vi "Dashboard Main.vi"() -> ()   [LabVIEW 2015]
uses:
  <vilib>/Utility/miscctls.llb/LVRowAndColumnTypeDef.ctl
  <vilib>/event_ctls.llb/eventvkey.ctl
  <vilib>/Rock Robotics/Network Tables/NT Read Numeric Array.vi
  <vilib>/Rock Robotics/WPI/Dashboard/WPI_DashboardLogging Global.vi
  Projects/FRC Operator Interface Control Board/controlBoard_LabVIEW/PWM_Output_TypeDef.ctl
  Projects/FRC Operator Interface Control Board/controlBoard_LabVIEW/LED_Output_TypeDef.ctl
  <vilib>/Rock Robotics/Network Tables/NT Write Raw.vi
  <vilib>/Rock Robotics/Network Tables/NT Read Raw.vi
panel:
  in  "TCP":refnum<k5>
  out "Image Message":string="Timeout in Camera Communications"
  in  "Dashboard Tab":T1(tab)
  out "Autonomous Selection":u8(ring) items=["Off", "Cross Defense", "Low Bar", "Cross Defense & Shoot", "Low Bar & Shoot"]
  out "Pneumatic Presure":u8(slide) scale=0.0..150.0
  out "Connected":bool
  out "COM Port":refnum<visa-resource-name>
  out "NT Connection":bool
  out "MotorChart R":cluster{"Numeric":dbl, "Numeric":dbl}(graph)
  out "MotorChart L":T2(graph)
  out "MotorSliders R":cluster{"MotorSlide1":dbl, "MotorSlide2":dbl} {"MotorSlide2" scale=-1.0..1.0 scale format="%#_2e"; "MotorSlide1" scale=-1.0..1.0 scale format="%#_2e"}
  out "MotorSliders L":T3 {"MotorSlide4 2" scale=0.0..14.0 scale format="%#_2e"; "MotorSlide2" scale=-1.0..1.0 scale format="%#_2e"; "MotorSlide1" scale=-1.0..1.0 scale format="%#_2e"}
  out "JS1 Z":dbl(slide) scale=-1.0..1.0 scale format="%#_2e"
  out "JS1 Graph":cluster{"X":dbl, "Y":dbl}[](graph)
  out "JS1 Buttons":T4
  out "JS2 Z":dbl(slide) scale=-1.0..1.0 scale format="%#_2e"
  out "JS2 Graph":cluster{"X":dbl, "Y":dbl}[](graph)
  out "JS2 Buttons":T4
  out "Mode":T5(ring)=enum."Auto Disabled"
  in  "DB Camera Config":bool
  out "fps":dbl format="%#.1g"
  out "Mbps":dbl format="%#.1g"
  out "Mbps LED":bool
  in  "Test Slider":dbl(slide) scale=0.0..100.0 scale format="%#_3g"
  in  "On/Off":bool caption="Solenoid"
  in  "Test Name":u16(ring) items=["Select the test to run..."]
  in  "Test Tree":string(tree)
  in  "Motor":cluster{"Value":dbl, "Enable":bool} {"Value" scale=-1.0..1.0 scale format="%#_3g"}
  out "Progress":T6 {"Test Progress" scale=0.0..100.0}
  in  "Rev/Fwd":cluster{"Forward":bool, "Reverse":bool}
  in  "Test Ring":u16(ring) items=["Monochrome", "Color"]
  out "Cmd Status":string
  in  "Execute Command":bool
  in  "Command Params":string[][](table)
  in  "Command Selection":i32(listbox)
  in  "CheckList":i32(listbox)
  out "Tree":string(tree)
  out "Camera Image":T7(plugin-control)
  # "Left"
  # "Front"
  # "Right"
  # "Battery"
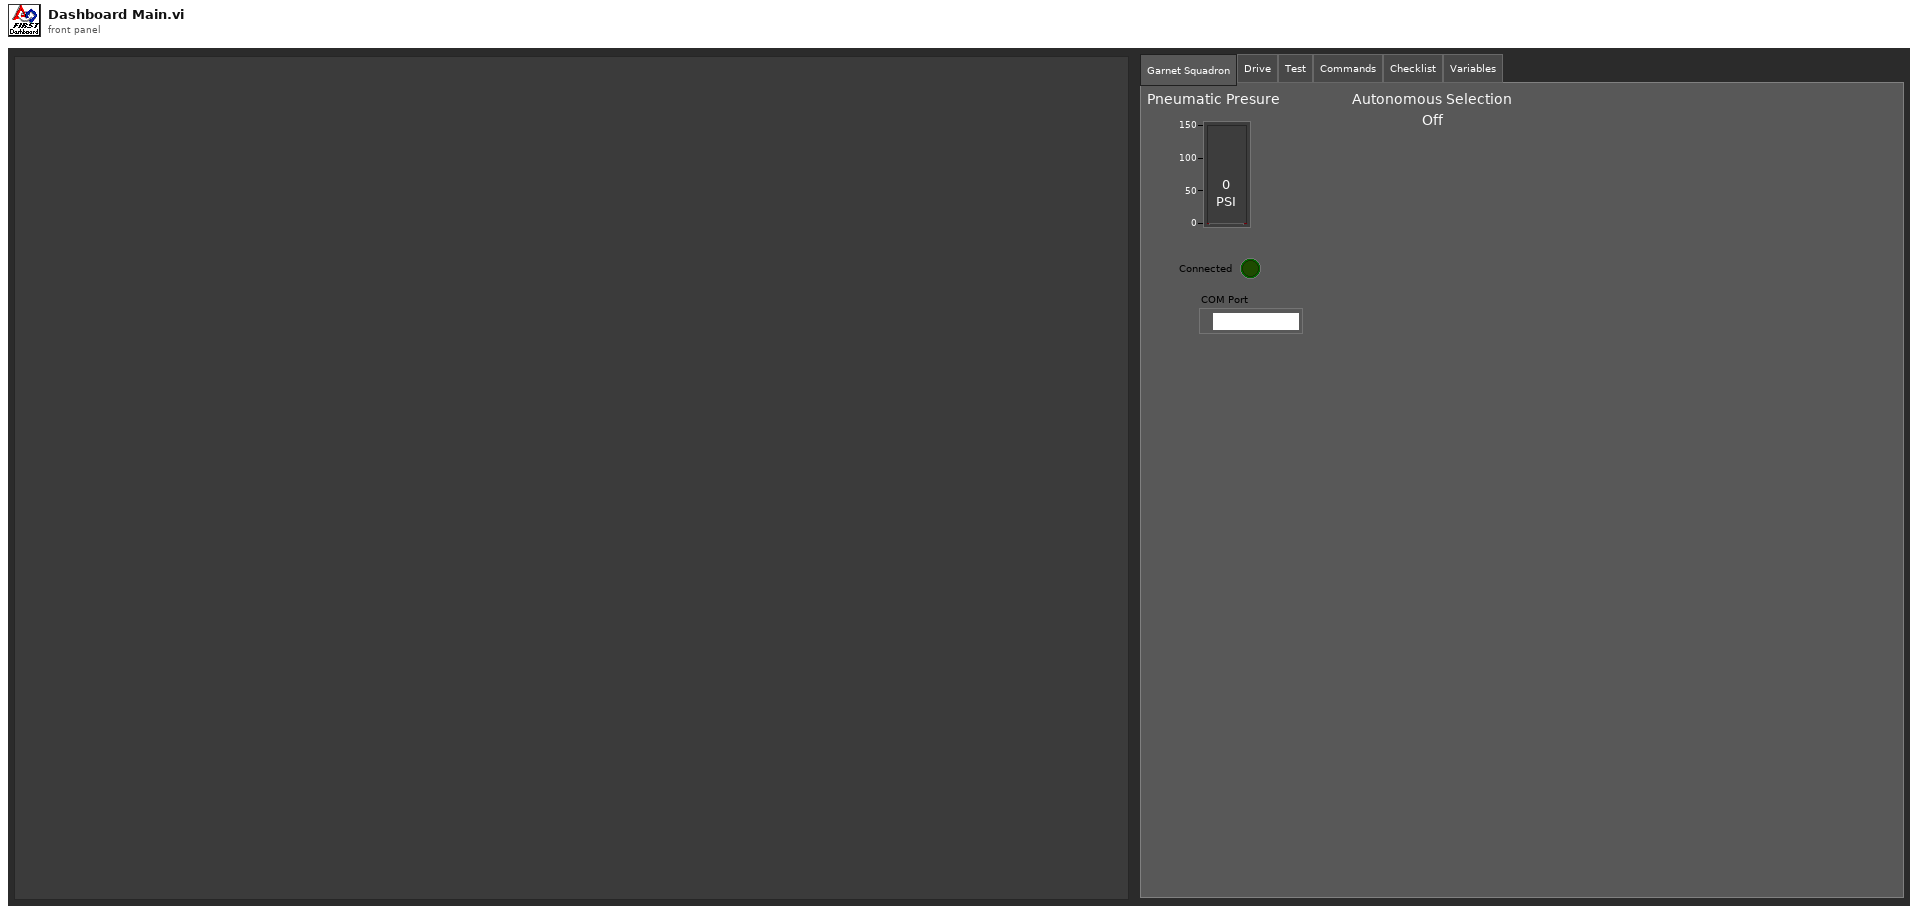
[diagram p1: front panel]
types:
  T1 = enum32{"Garnet Squadron", "Drive", "Test", "Commands", "Checklist", "Variables"}
  T2 = cluster{"Numeric":dbl, "Numeric":dbl, "Battery V":dbl}
  T3 = cluster{"MotorSlide1":dbl, "MotorSlide2":dbl, "MotorSlide4 2":dbl}
  T4 = cluster{bool, bool, bool, bool, bool, bool, bool, bool, bool, bool, bool, bool}
  T5 = enum8{"Tele-Op Disabled", "Tele-Op Enabled", "Auto Disabled", "Auto Enabled", "Test Disabled", "Test Enabled", "Disconnected", "No Code", "E-Stop"}
  T6 = cluster{"Test Progress":u8, "Test Progress Text":string}
  T7 = typedef "IMAQ Image.ctl" = refnum<image>
  T8 = enum8{"Enabled", "Disabled", "Disabled and Grayed Out"}
  T9 = cluster{"IDs":cluster{"RPC field ID":u16, "Unique ID":u16}, "String":string}
  T10 = enum32{"Drive", "Basic", "Custom", "Test", "Checklist", "Variables"}
  T11 = typedef "Image Type" = u32
  T12 = typedef "LED_Output_TypeDef.ctl" = cluster{"LED 0":bool, "LED 1":bool, "LED 2":bool, "LED 3":bool, "LED 4":bool, "LED 5":bool, "LED 6":bool, "LED 7":bool, "LED 8":bool, "LED 9":bool, "LED 10":bool, "LED 11":bool, "LED 12":bool, "LED 13":bool, "LED 14":bool, "LED 15":bool}
  T13 = typedef "PWM_Output_TypeDef.ctl" = cluster{"PWM 0":u8, "PWM 1":u8, "PWM 2":u8, "PWM 3":u8, "PWM 4":u8, "PWM 5":u8, "PWM 6":u8, "PWM 7":u8, "PWM 8":u8, "PWM 9":u8, "PWM 10":u8}
  T14 = typedef "Analog_Input_TypeDef.ctl" = cluster{"ANA 0":u8, "ANA 1":u8, "ANA 2":u8, "ANA 3":u8, "ANA 4":u8, "ANA 5":u8, "ANA 6":u8, "ANA 7":u8, "ANA 8":u8, "ANA 9":u8, "ANA 10":u8, "ANA 11":u8, "ANA 12":u8, "ANA 13":u8, "ANA 14":u8, "ANA 15":u8}
  T15 = typedef "Switch_Input_TypeDef.ctl" = cluster{"SW 0":bool, "SW 1":bool, "SW 2":bool, "SW 3":bool, "SW 4":bool, "SW 5":bool, "SW 6":bool, "SW 7":bool, "SW 8":bool, "SW 9":bool, "SW 10":bool, "SW 11":bool, "SW 12":bool, "SW 13":bool, "SW 14":bool, "SW 15":bool}
  T16 = cluster{"Error Strings":string, "Disable Counts":cluster{u16, u16}, "Rail Faults":cluster{u16, u16, u16}, "Robot IP":string, "DB Mode":u8, "Event Info":cluster{"Name":string, "Type":u8, "Number":u16, "Replay":u8}, "Camera Addr":string}
  T17 = cluster{"Storage":cluster{"Disk Free":u64, "RAM Block":u32, "RAM free":u32}, "CPU Utilization":cluster{"CPU % ISR":sgl, "CPU % Time Crit":sgl, "CPU % Timed Str":sgl, "CPU % High":sgl, "CPU % Above":sgl, "CPU % Normal":sgl, "CPU % Low":sgl}, "CAN":cluster{"% Bus Utilization":sgl, "Bus Off Cnt":u32, "TX_FIFO Full Cnt":u32, "Receive Error Cnt":u8, "Transmit Error Cnt":u8}, "HID":cluster{"HID Outputs":u32, "Rumble Low":u16, "Rumble High":u16}[]}
  T18 = cluster{"Status bits":cluster{"Test Mode":bool, "Autonomous":bool, "Enabled":bool, "Code Start":bool, "Brownout":bool, "Reserved 2":bool, "Reserved 3":bool, "E-Stop":bool}, "Code Trace":cluster{"Disabled":bool, "TeleOp":bool, "Auto":bool, "Test":bool}, "Controller Type":enum16{"unknown", "cRIO", "roboRio"}, "Code?":enum16{"unknown", "noCode", "code"}, "Battery V":dbl}
  T19 = cluster{"Control Bits":cluster{"TestMode":bool, "Autonomous":bool, "Enabled":bool, "FMS Present":bool, bool, bool, bool, "E-Stop":bool}, "Team Station ":u8, "Countdown":sgl, "Joystick Values":cluster{"Axes":dbl[], "Buttons":bool[], "POVs":i16[]}[]}
  T20 = cluster{"Axes":dbl[], "Buttons":bool[], "POVs":i16[]}[]
  T21 = cluster{"Axes":dbl[], "Buttons":bool[], "POVs":i16[]}
  T22 = cluster{"Buttons[0]":bool, "Buttons[1]":bool, "Buttons[2]":bool, "Buttons[3]":bool, "Buttons[4]":bool, "Buttons[5]":bool, "Buttons[6]":bool, "Buttons[7]":bool, "Buttons[8]":bool, "Buttons[9]":bool, "Buttons[10]":bool, "Buttons[11]":bool}
  T23 = typedef "NI_LVConfig.lvlib/Config Data RefNum.ctl" = refnum<k1>
  T24 = cluster{"Operation":enum16{"Update", "Clear"}, "Color Box":u32}[]
  T25 = typedef "eventvkey.ctl" = enum16{"ASCII", "Enter", "Return", "Shift", "Ctrl", "Alt", "Cmd", "Opt", "Caps", "NumLock", "Clear", "Break", "Up", "Down", "Left", "Right", "Insert", "Delete", "Home", "End", "PageUp", "PageDown", "Escape", "Help", "Pause", "ScrollLock", "F1", "F2", "F3", "F4", "F5", "F6", "F7", "F8", "F9", "F10", "F11", "F12", "F13", "F14", "F15", "F16", "F17", "F18", "F19", "F20", "F21", "F22", "F23", "F24", "Play", "VolumeUp", "VolumeDown", "Mute", "Two Byte Char"}
  T26 = cluster{"Operation":enum16{"Update", "Clear"}, "Color Box":u32}
  T27 = typedef "LVRowAndColumnTypeDef.ctl" = cluster{"Row":i32, "Column":i32}
  T28 = cluster{"Shift":bool, "Ctrl":bool, "Alt":bool, "Cmd":bool, "Opt":bool}
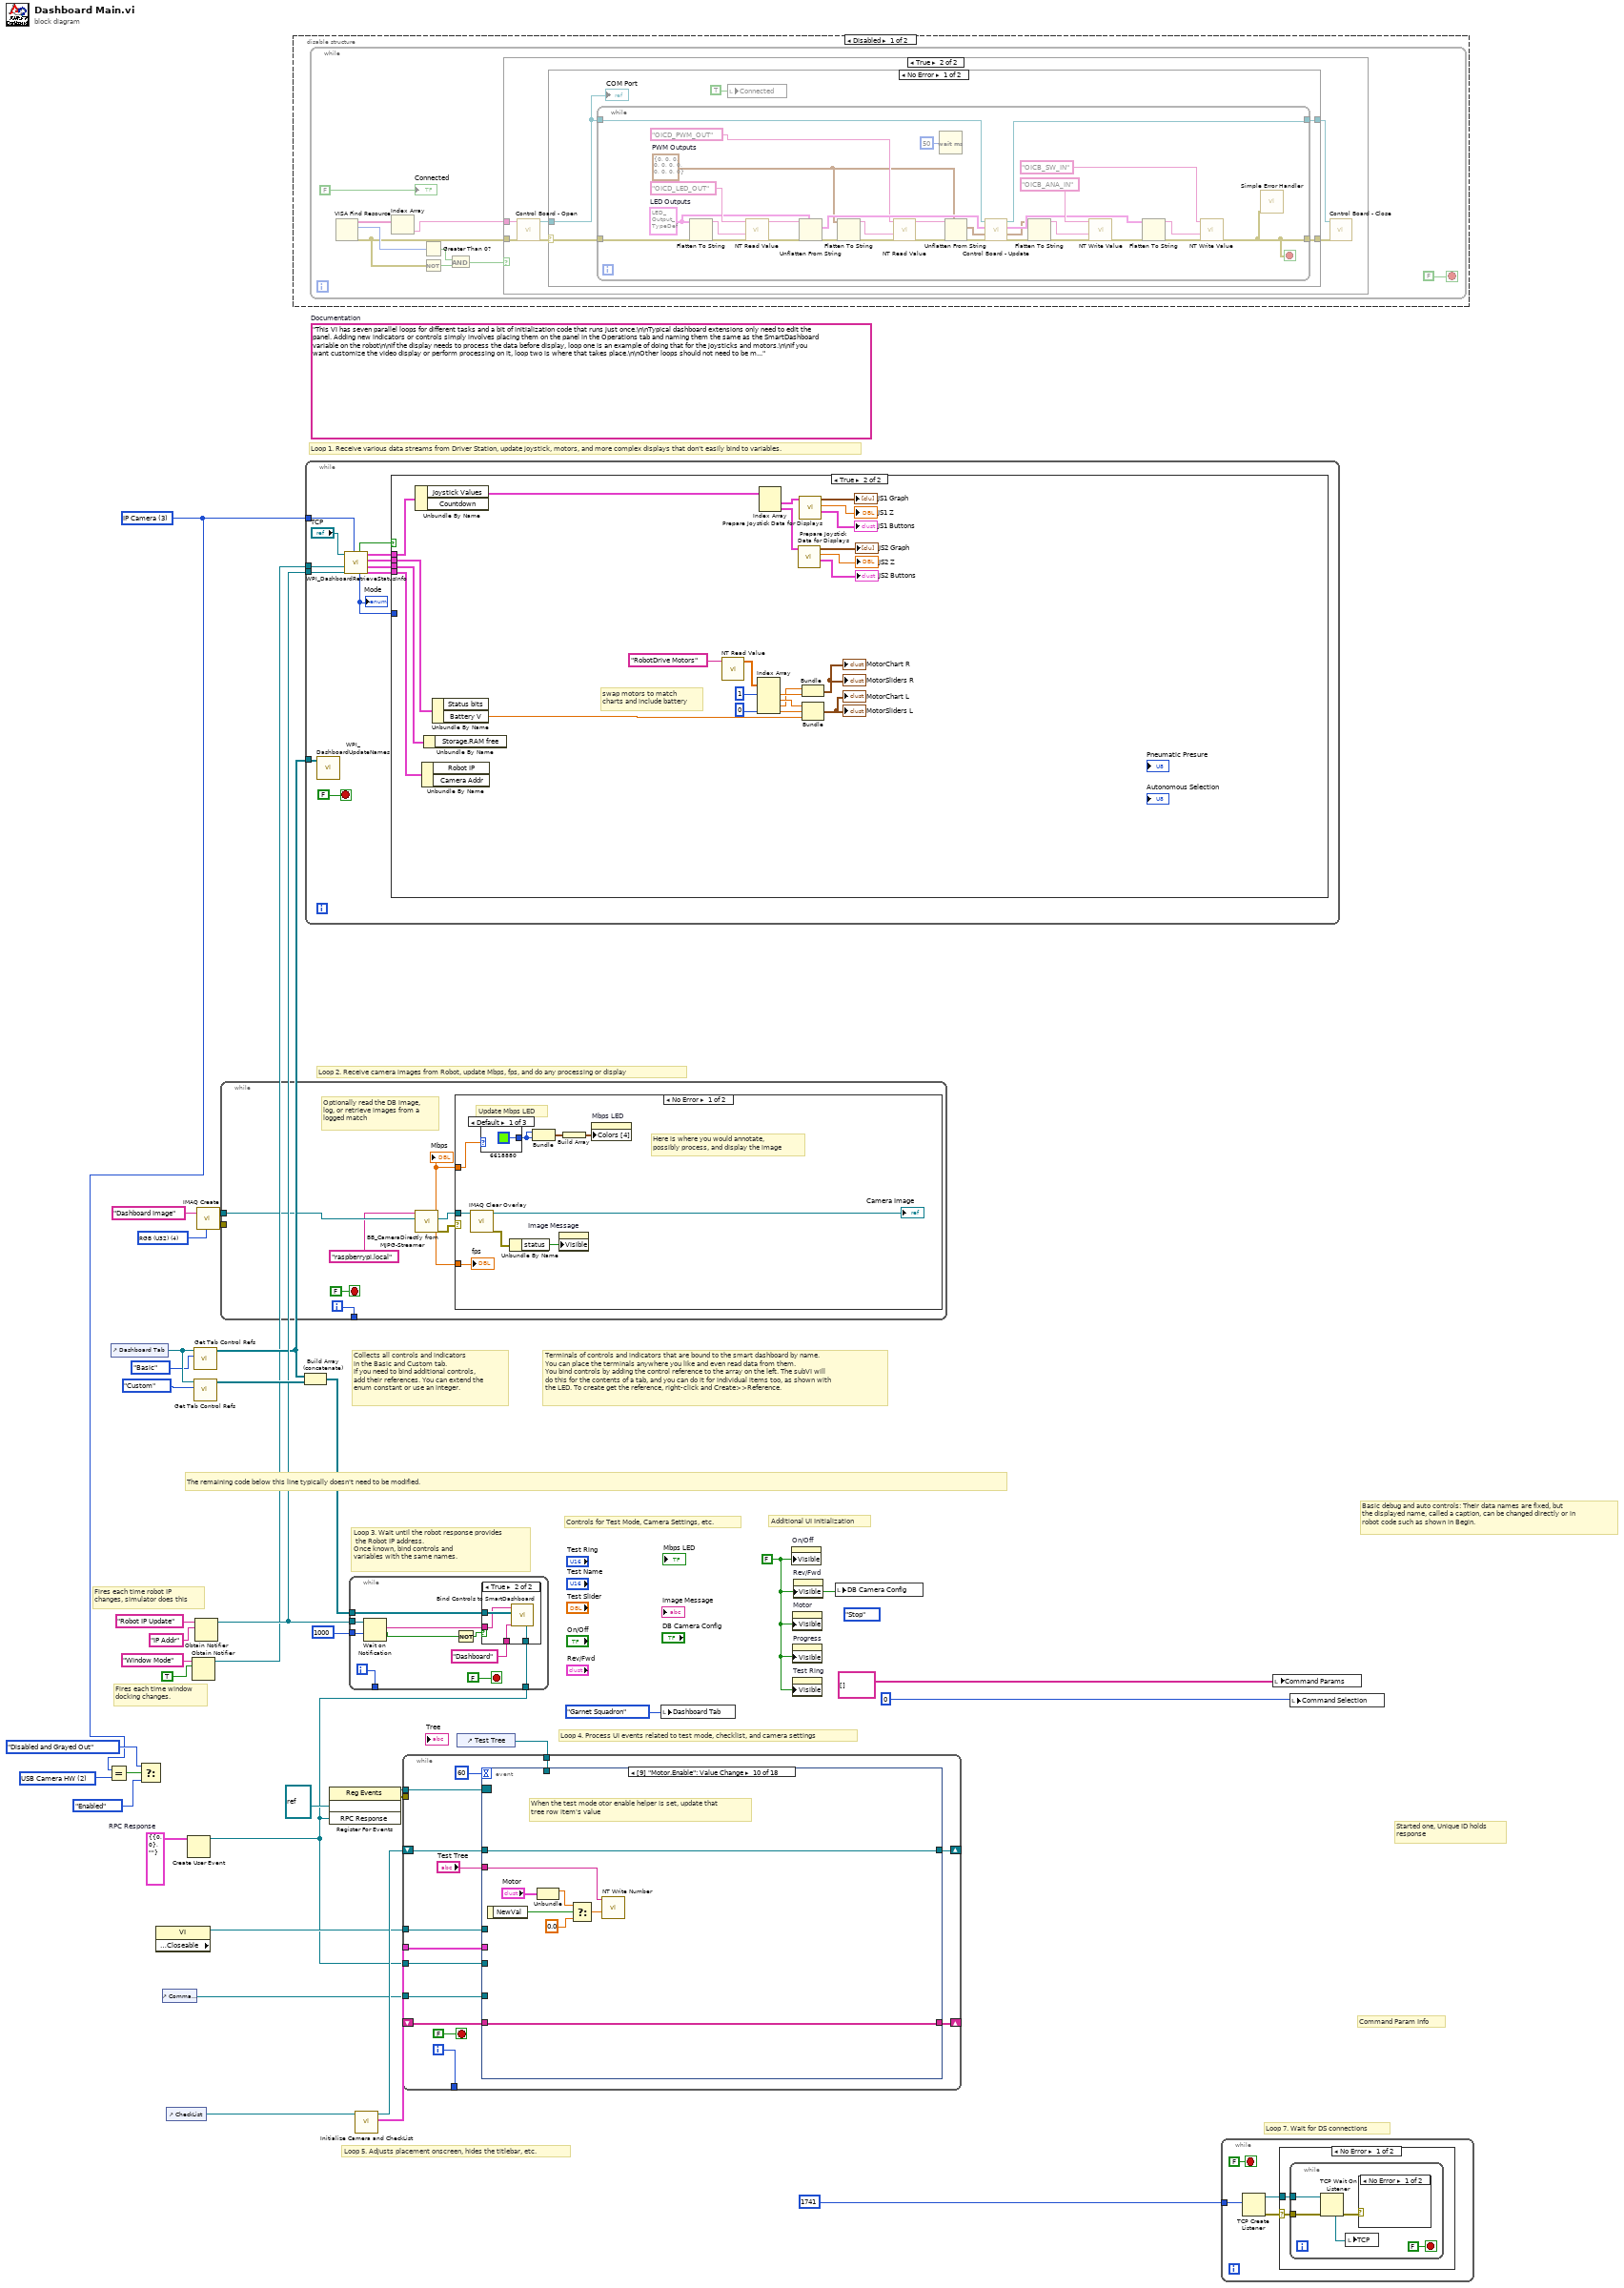
[diagram p0: block diagram]
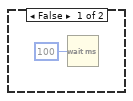
[diagram p2: hidden frame]
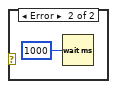
[diagram p5: hidden frame]
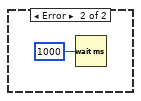
[diagram p6: hidden frame]
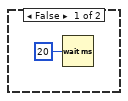
[diagram p7: hidden frame]
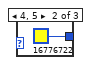
[diagram p9: hidden frame]
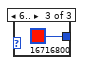
[diagram p10: hidden frame]
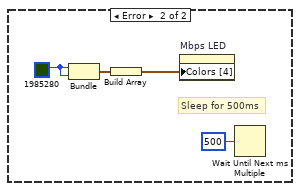
[diagram p11: hidden frame]
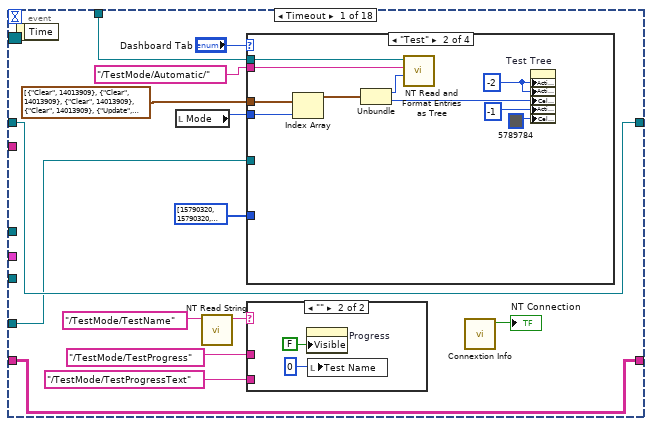
[diagram p12: hidden frame]
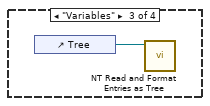
[diagram p14: hidden frame]
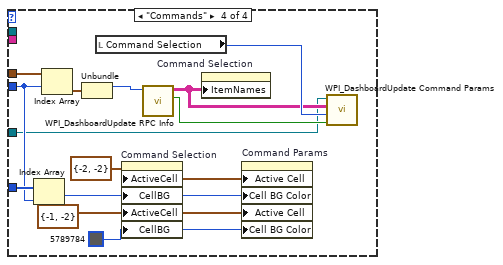
[diagram p15: hidden frame]
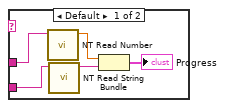
[diagram p16: hidden frame]
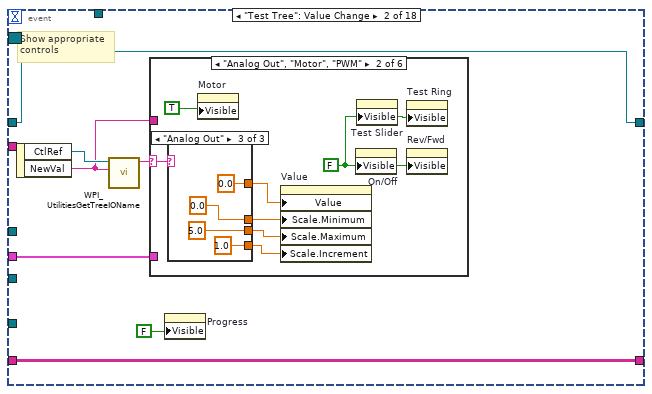
[diagram p17: hidden frame]
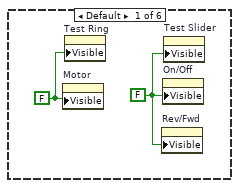
[diagram p18: hidden frame]
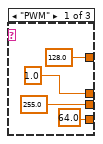
[diagram p19: hidden frame]
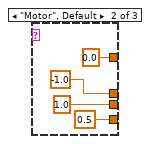
[diagram p20: hidden frame]
diagram:
  w1 = u16 2 items=["Camera Off", "USB Camera SW", "USB Camera HW", "IP Camera"] ("Vision")
  w2 = u16 3 items=["Camera Off", "USB Camera SW", "USB Camera HW", "IP Camera"] ("Vision")
  w10 = T9 {"IDs"={"RPC field ID"=0, "Unique ID"=0}, "String"=""}  # RPC Response
  (unwired) enum32{"Stop", "Record", "Playback"}."Stop" ("Rec Mode")
  w16 = FALSE ("Visible")
  (unwired) "This VI has seven parallel loops for different tasks and a bit of initialization code that runs just once.\n\nTypical dashboard extensions only need to edit the panel. Adding new indicators or controls simply involves placing them on the panel in the Operations tab and naming them the same as the SmartDashboard variable on the robot\n\nIf the display needs to process the data before display, loop one is an example of doing that for the joysticks and motors.\n\nIf you want customize the video display or perform processing on it, loop two is where that takes place.\n\nOther loops should not need to be modified. They are pretty standard, and document the task they perform."  # Documentation
  w38 = T11 4 items=["Grayscale (U8)", "Grayscale (I16)", "Grayscale (SGL)", "Complex (CSG)", "RGB (U32)", "HSL (U32)", "RGB (U64)"] ("Image Type")
  # "Command Param Info"
  # "Started one, Unique ID holds\nresponse"
  # "Loop 7. Wait for DS connections"
  # "Basic debug and auto controls: Their data names are fixed, but\nthe displayed name, called a caption, can be changed directly or in\nrobot code such as shown in Begin."
  # "Controls for Test Mode, Camera Settings, etc."
  # "Additional UI Initialization"
  # "Fires each time robot IP\nchanges, simulator does this"
  # "Fires each time window\ndocking changes."
  # "Collects all controls and indicators\nin the Basic and Custom tab.\nIf you need to bind additional controls,\nadd their references. You can extend the\nenum constant or use an integer."
  # "The remaining code below this line typically doesn't need to be modified."
  # "Loop 4. Process UI events related to test mode, checklist, and camera settings"
  # "Terminals of controls and indicators that are bound to the smart dashboard by name.\nYou can place the terminals anywhere you like and even read data from them.\nYou bind controls by adding the control reference to the array on the left. The subVI will\ndo this for the contents of a tab, and you can do it for individual items too, as shown with\nthe LED. To create get the reference, right-click and Create>>Reference."
  # "Loop 3. Wait until the robot response provides\n the Robot IP address.\nOnce known, bind controls and\nvariables with the same names."
  # "Loop 5. Adjusts placement onscreen, hides the titlebar, etc."
  # "Loop 1. Receive various data streams from Driver Station, update joystick, motors, and more complex displays that don't easily bind to variables."
  # "Loop 2. Receive camera images from Robot, update Mbps, fps, and do any processing or display"
  n1 = Equal?(x=w2, y=w1) -> (x = y?=w5:bool)
  n2 = control-ref of="Dashboard Tab"() -> (w22:refnum<vi>)
  n3 = Select(t=T8."Disabled and Grayed Out" ("Disabled"), s=w5, f=T8."Enabled" ("Disabled")) -> ()  [unwired: 1 out]
  n4 = property class="VI" props=["Front Panel.Closeable"]() -> (reference out=w23:refnum<vi>)  [unwired: 2 in, 2 out]
  n5 = control-ref of="Command Params"() -> (w6:refnum<vi>)
  n6 = control-ref of="CheckList"() -> (w17:refnum<vi>)
  n7 = Create User Event(user event datatype=w10) -> (user event=w7:refnum<user-event>)  [unwired: 1 in, 1 out]
  n8 = Obtain Notifier(name (unnamed)="Window Mode", notification data type=TRUE) -> (notifier out=w13:refnum<notifier>)  [unwired: 2 in, 2 out]
  n9 = call <vilib>:"Get Tab Control Refs.vi"("Page Index"=T10."Basic" ("Dashboard Tab"), "TabControl in"=w22) -> ("ControlsOnPage"=w14:refnum<vi>[])  [unwired: 9 in]
  n10 = call <vilib>:"Get Tab Control Refs.vi"("Page Index"=T10."Custom" ("Dashboard Tab"), "TabControl in"=w22) -> ("ControlsOnPage"=w21:refnum<vi>[])  [unwired: 9 in]
  n11 = Obtain Notifier(name (unnamed)="Robot IP Update", notification data type="IP Addr" ("name (unnamed)")) -> (notifier out=w15:refnum<notifier>)  [unwired: 2 in, 2 out]
  n12 = call "IMAQ Create"("Image Name"="Dashboard Image", "Image Type"=w38) -> ("New Image"=w36:T7, "error out"=w35:errorcluster)  [unwired: 2 in, 1 out]
  n13 = while {
    tunnel: w36 -> [w44]
    tunnel: w35 -> [_]
    tunnel: [w45] -> _
    i -> [w45]
    stop <- FALSE stop-if-true
    # "Optionally read the DB image,\nlog, or retrieve images from a\nlogged match"
    n14 = call "BB_CameraDirectly from MJPG-Streamer.vi"("Image"=w44, "address"="raspberrypi.local" ("Camera IP")) -> ("error out"=w42:errorcluster, "Bandwidth (Mbps)"=w40:dbl, "Image Out"=w43:T7, "FPS"=w41:dbl)  [unwired: 6 in]
    "Mbps" <- w40
    n15 = case shown="No Error" w42 {
      tunnel: w43 -> [w50 _]
      tunnel: w40 -> [w49 _]
      tunnel: w41 -> [w47 _]
      frame No Error {
        # "Here is where you would annotate,\npossibly process, and display the image"
        # "Update Mbps LED"
        n16 = call "IMAQ Clear Overlay"("Image"=w50) -> ("error out"=w54:errorcluster, "Image Out"=→"Camera Image":T7)  [unwired: 2 in, 7 out]
        n17 = case shown="Default" w49 {
          tunnel: [u32 6618880 ("Color Box") u32 16776722 ("Color Box") u32 16716800 ("Color Box")] -> w51
          frame Default {
          }
          frame 4, 5 {
          }
          frame 6.. {
          }
        }
        n18 = Unbundle By Name(w54) -> ("status"=w55:bool)
        n19 = Bundle("Color Box"=w51, "Color Box"=w51) -> (w53:cluster{"Color Box":u32, "Color Box":u32})  [unwired: 1 out]
        n20 = property on="Image Message" class="Str"("Visible"=w55) -> ()  [unwired: 2 in, 2 out]
        n21 = Build Array(w53) -> (w52:cluster{"Color Box":u32, "Color Box":u32}[])
        n22 = property on="Mbps LED" class="Bool (strict)"("Colors [4]"=w52) -> ()  [unwired: 2 in, 2 out]
        "fps" <- w47
      }
      frame Error {
        w59 = u32 1985280 ("Color Box")
        # "Sleep for 500ms"
        n23 = Bundle("Color Box"=w59, "Color Box"=w59) -> (w61:cluster{"Color Box":u32, "Color Box":u32})  [unwired: 1 out]
        n24 = Build Array(w61) -> (w60:cluster{"Color Box":u32, "Color Box":u32}[])
        n25 = property on="Mbps LED" class="Bool (strict)"("Colors [4]"=w60) -> ()  [unwired: 2 in, 2 out]
        n26 = Wait Until Next ms Multiple(millisecond multiple=u32 500) -> ()  [unwired: 1 out]
      }
    }
  }
  n27 = disable-structure shown="Disabled" {
    frame Disabled {
      n28 = while {
        stop <- FALSE stop-if-true
        n29 = VISA Find Resource() -> (0:w65:errorcluster, 2:w71:u32, 3:w70:string[])  [unwired: 3 in]
        n30 = Index Array(array=w70) -> (element=w69:string)  [unwired: 1 in]
        n31 = Greater Than 0?(x=w71) -> (x > 0?=w68:bool)
        n32 = Not(x=w65) -> (.not. x?=w66:bool)
        n33 = And(x=w68, y=w66) -> (x .and. y?=w67:bool)
        n34 = case shown="True" w67 {
          tunnel: w69 -> [_ w77]
          tunnel: w65 -> [_ w76]
          frame False {
            n35 = Wait (ms)(milliseconds to wait=u32 100) -> ()  [unwired: 1 out]
          }
          frame True {
            n36 = call "Control Board - Open.vi"("error in (no error)"=w76, "VISA Refnum in"=w77) -> ("error out"=w75:errorcluster, "VISA Refnum out"=w78:refnum<visa-resource-name>)  [unwired: 8 in]
            n37 = case shown="No Error" w75 {
              selector: w75 -> [w82 w116]
              tunnel: w78 -> [w83 w115]
              tunnel: [w80 w116] -> w74
              tunnel: [w79 w115] -> w73
              frame No Error {
                n38 = while {
                  tunnel: w83 -> [w114]
                  tunnel: [w112] -> w79
                  tunnel: [w84] -> w80
                  tunnel: w82 -> [w86]
                  stop <- w84 stop-if-true
                  w93 = T12 {"LED 0"=FALSE, "LED 1"=FALSE, "LED 2"=FALSE, "LED 3"=FALSE, "LED 4"=FALSE, "LED 5"=FALSE, "LED 6"=FALSE, "LED 7"=FALSE, "LED 8"=FALSE, "LED 9"=FALSE, "LED 10"=FALSE, "LED 11"=FALSE, "LED 12"=FALSE, "LED 13"=FALSE, "LED 14"=FALSE, "LED 15"=FALSE}  # LED Outputs
                  w91 = T13 {"PWM 0"=0, "PWM 1"=0, "PWM 2"=0, "PWM 3"=0, "PWM 4"=0, "PWM 5"=0, "PWM 6"=0, "PWM 7"=0, "PWM 8"=0, "PWM 9"=0, "PWM 10"=0}  # PWM Outputs
                  n39 = Flatten To String(anything=w93, error in (no error)=w86) -> (data string=w92:string, error out=w87:errorcluster)  [unwired: 2 in, 1 out]
                  n40 = call-poly <vilib>:"NT Read Value.vi"("error in"=w87, "Default Value"=w92, "Name"="OICD_LED_OUT") -> ("error out"=w100:errorcluster, "Raw"=w102:string)  [unwired: 7 in]
                  n41 = Unflatten From String(type=w93, binary string=w102, error in (no error)=w100) -> (value=w104:T12, error out=w88:errorcluster)  [unwired: 2 in, 1 out]
                  n42 = Flatten To String(anything=w91, error in (no error)=w88) -> (data string=w90:string, error out=w89:errorcluster)  [unwired: 2 in, 1 out]
                  n43 = call-poly <vilib>:"NT Read Value.vi"("error in"=w89, "Default Value"=w90, "Name"="OICD_PWM_OUT") -> ("error out"=w95:errorcluster, "Raw"=w108:string)  [unwired: 7 in]
                  n44 = Wait (ms)(milliseconds to wait=u32 50) -> ()  [unwired: 1 out]
                  n45 = Unflatten From String(type=w91, binary string=w108, error in (no error)=w95) -> (value=w107:T13, error out=w94:errorcluster)  [unwired: 2 in, 1 out]
                  n46 = call "Control Board - Update.vi"("error in (no error)"=w94, "PWM Outputs"=w107, "LED Outputs"=w104, "Control Board VISA Reference In"=w114) -> ("error out"=w97:errorcluster, "Analog Inputs"=w106:T14, "Switch Inputs"=w110:T15, "Control Board VISA Reference Out"=w112:refnum<visa-resource-name>)  [unwired: 4 in]
                  n47 = Flatten To String(anything=w106, error in (no error)=w97) -> (data string=w105:string, error out=w99:errorcluster)  [unwired: 2 in, 1 out]
                  n48 = call-poly <vilib>:"NT Write Value.vi"("error in"=w99, "Raw"=w105, "Name"="OICB_ANA_IN") -> ("error out"=w96:errorcluster)  [unwired: 8 in]
                  n49 = Flatten To String(anything=w110, error in (no error)=w96) -> (data string=w109:string, error out=w98:errorcluster)  [unwired: 2 in, 1 out]
                  n50 = call-poly <vilib>:"NT Write Value.vi"("error in"=w98, "Raw"=w109, "Name"="OICB_SW_IN") -> ("error out"=w84:errorcluster)  [unwired: 8 in]
                  n51 = call <vilib>:"Simple Error Handler.vi"("error in (no error)"=w84) -> ()  [unwired: 4 in, 5 out]
                }
                n52 = local write "Connected"(TRUE ("Connected")) -> ()
                "COM Port" <- w83
              }
              frame Error {
              }
            }
            n53 = call "Control Board - Close.vi"("error in (no error)"=w74, "VISA Refnum in"=w73) -> ()  [unwired: 9 in, 1 out]
          }
        }
        "Connected" <- FALSE
      }
    }
    frame Enabled {
    }
  }
  n54 = Build Array (concatenate)(w14, w21) -> (w20:refnum<vi>[])
  n55 = while {
    tunnel: w15 -> [w122]
    tunnel: w14 -> [w121]
    tunnel: w13 -> [w118]
    tunnel: w2 -> [w117]
    stop <- FALSE stop-if-true
    n56 = call <vilib>:"WPI_DashboardUpdateNames.vi"("Controls on Tab"=w121) -> ()  [unwired: 11 in]
    n57 = call <vilib>:"WPI_DashboardRetrieveStatusInfo.vi"("Vision"=w117, "Binding Refnum"=w122, "Window Mode Notifier"=w118, "TCP Cnx"="TCP") -> ("Power and Errors"=w123:T16, "Robot Metrics"=w126:T17, "Status Info"=w127:T18, "Control Info"=w124:T19, "Robot Mode"=w120:T5, "Process?"=w125:bool)  [unwired: 2 in]
    "Mode" <- w120
    n58 = case shown="True" w125 {
      tunnel: w127 -> [_ w153]
      tunnel: w126 -> [_ w152]
      tunnel: w124 -> [_ w151]
      tunnel: w123 -> [_ w150]
      tunnel: w120 -> [_ _]
      frame False {
        n59 = Wait (ms)(milliseconds to wait=u32 20) -> ()  [unwired: 1 out]
      }
      frame True {
        # "swap motors to match\ncharts and include battery"
        n60 = Unbundle By Name(w151) -> ("Joystick Values"=w140:T20)  [unwired: 1 out]
        n61 = Unbundle By Name(w150) -> ()  [unwired: 2 out]
        n62 = Unbundle By Name(w152) -> ()  [unwired: 1 out]
        n63 = Unbundle By Name(w153) -> ("Battery V"=w141:dbl)  [unwired: 1 out]
        n64 = call-poly <vilib>:"NT Read Value.vi"("Name"="RobotDrive Motors") -> ("Numeric Array"=w130:dbl[])  [unwired: 9 in, 1 out]
        n65 = Index Array(array=w130, index #1=1, index #4=0) -> (element #1=w145:dbl, element #2=w146:dbl, element #3=w144:dbl, element #4=w149:dbl)  [unwired: 2 in]
        n66 = Index Array(array=w140) -> (element #1=w139:T21, element #2=w135:T21)  [unwired: 2 in]
        n67 = call "Prepare Joystick Data for Displays.vi"("Joystick Values"=w135) -> ("Buttons"=→"JS2 Buttons":T22, "Z Axis"=→"JS2 Z":dbl, "Cartesian Data"=→"JS2 Graph":cluster{"X axis":dbl, "X axis":dbl}[])  [unwired: 8 in]
        n68 = call "Prepare Joystick Data for Displays.vi"("Joystick Values"=w139) -> ("Buttons"=→"JS1 Buttons":T22, "Z Axis"=→"JS1 Z":dbl, "Cartesian Data"=→"JS1 Graph":cluster{"X axis":dbl, "X axis":dbl}[])  [unwired: 8 in]
        n69 = Bundle("Numeric"=w144, "Numeric"=w145) -> (→"MotorChart R" →"MotorSliders R":cluster{"Numeric":dbl, "Numeric":dbl})  [unwired: 1 in]
        n70 = Bundle("Numeric"=w146, "Numeric"=w149, "Battery V"=w141) -> (→"MotorChart L" →"MotorSliders L":T2)  [unwired: 1 in]
      }
    }
  }
  n71 = register-events(refnum<vi> refnum, w7) -> (reference out=w27:refnum<event-registration>, error out=w26:errorcluster)  [unwired: 2 in]
  n72 = while {
    tunnel: w20 -> [w163]
    tunnel: w15 -> [w161]
    tunnel: [w159] -> _
    tunnel: u32 1000 ("milliseconds to wait") -> [w158]
    tunnel: w7 -> [w154]
    i -> [w159]
    stop <- FALSE stop-if-true
    n73 = Wait on Notification(notifier=w161, timeout in ms (-1)=w158) -> (notification=w160:string, timed out?=w156:bool)  [unwired: 2 in, 2 out]
    n74 = Not(x=w156) -> (.not. x?=w157:bool)
    n75 = case shown="True" w157 {
      tunnel: w163 -> [_ w167]
      tunnel: w160 -> [_ w166]
      tunnel: "Dashboard" -> [_ w165]
      tunnel: w154 -> [_ w164]
      frame False {
      }
      frame True {
        n76 = call <vilib>:"Bind Controls to SmartDashboard.vi"("RPC ref"=w164, "Client Name"=w165, "Bound Control Refs"=w167, "Server IP Address"=w166) -> ()  [unwired: 8 in]
      }
    }
  }
  n77 = call "Initialize Camera and CheckList.vi"("ListBox in"=w17) -> ("Array"=w30:cluster{string[]}[], "File Refnum"=w29:T23)  [unwired: 8 in, 1 out]
  n78 = control-ref of="Test Tree"() -> (w28:refnum<vi>)
  n79 = while {
    tunnel: w30 -> [w178]
    shift-right: [w177] -> _
    shift-left: w29 -> [w176]
    tunnel: [w175] -> _
    tunnel: w28 -> [w174]
    tunnel: w27 -> [w173]
    tunnel: w26 -> [_]
    tunnel: w23 -> [w172]
    tunnel: w7 -> [w171]
    tunnel: w6 -> [w170]
    shift-right: [w169] -> _
    shift-left: _ -> [w168]
    i -> [w175]
    stop <- FALSE stop-if-true
    n80 = event shown="[9] \"Motor.Enable\": Value Change" {
      selector: w173 -> [_ _ _ _ _ _ _ _ _ _ _ _ _ _ _ _ _ _]
      dyn-events: _ -> [_ _ _ _ _ _ _ _ _ _ _ _ _ _ _ _ _ _]
      timeout: u32 60 ("milliseconds to wait") -> [_ _ _ _ _ _ _ _ _ _ _ _ _ _ _ _ _ _]
      tunnel: w174 -> [w191 _ _ _ _ _ _ _ _ _ _ _ _ _ _ _ _ _]
      tunnel: "Test Tree" -> [_ _ _ _ _ _ _ _ _ w403 w412 w415 w420 w429 _ _ _ _]
      tunnel: w178 -> [_ w229 _ _ _ _ _ _ _ _ _ _ _ _ _ _ _ _]
      tunnel: [w188 w228 w332 w338 w350 w362 w370 w376 w389 w402 w410 w414 w419 w428 w435 w437 w444 w452] -> w177
      tunnel: w176 -> [w188 w228 w332 w338 w350 w362 w370 w376 w389 w402 w410 w414 w419 w428 w435 w437 w444 w452]
      tunnel: w172 -> [_ _ _ _ _ _ _ _ _ _ _ _ _ _ _ _ _ _]
      tunnel: w171 -> [_ _ _ _ _ _ _ _ _ _ _ _ _ _ _ _ _ _]
      tunnel: w170 -> [w183 _ _ _ w348 _ _ _ _ _ _ _ _ _ _ _ _ _]
      tunnel: [w182 w227 w331 w337 w346 w356 w367 w375 w388 w401 w409 w413 w418 w427 w433 w436 w440 w453] -> w169
      tunnel: w168 -> [w182 w227 w331 w337 w346 _ _ w375 w388 w401 w409 w413 w418 w427 w433 w436 w440 w453]
      event Timeout {
        n81 = event-data() -> ()  [unwired: 1 in, 1 out]
        n82 = local read "Mode"() -> (w185:T5)
        n83 = call <vilib>:"NT Read String.vi"("Name"="/TestMode/TestName") -> ("String"=w194:string)  [unwired: 9 in, 1 out]
        n84 = case shown="\"Test\"" "Dashboard Tab" {
          tunnel: w191 -> [_ w205 _ _]
          tunnel: "/TestMode/Automatic/" ("Name Pattern") -> [_ w204 _ _]
          tunnel: T24 [{"Operation"=enum."Clear", "Color Box"=14013909}, {"Operation"=enum."Clear", "Color Box"=14013909}, {"Operation"=enum."Clear", "Color Box"=14013909}, {"Operation"=enum."Clear", "Color Box"=14013909}, {"Operation"=enum."Update", "Color Box"=14013909}, {"Operation"=enum."Update", "Color Box"=16777215}, {"Operation"=enum."Clear", "Color Box"=14013909}, {"Operation"=enum."Clear", "Color Box"=14013909}, {"Operation"=enum."Clear", "Color Box"=14013909}] -> [_ w197 _ w214]
          tunnel: w185 -> [_ w196 _ w213]
          tunnel: u32[] [15790320, 15790320, 15790320, 15790320, 16777215, 16777215, 15790320, 15790320, 15790320] -> [_ _ _ w219]
          tunnel: w183 -> [_ _ _ w207]
          frame "Garnet Squadron", Default {
          }
          frame "Test" {
            w203 = -2 ("Active Item:Row Number")
            n85 = Index Array(array=w197, index=w196) -> (element=w198:T26)
            n86 = Unbundle(w198) -> ("Operation"=w199:enum16{"Update", "Clear"}, "Color Box"=w200:u32)
            n87 = call <vilib>:"NT Read and Format Entries as Tree.vi"("Operation"=w199, "Name Pattern"=w204, "Tree Refnum"=w205) -> ()  [unwired: 7 in, 2 out]
            n88 = property on="Test Tree" class="Tree (strict)"("Active Item Row Number"=w203, "ActiveColNum"=w203, "CellBG"=w200, "Active Item Row Number"=-1 ("Active Item:Row Number"), "CellBG"=u32 5789784 ("Color Box")) -> ()  [unwired: 2 in, 2 out]
          }
          frame "Variables" {
            n89 = control-ref of="Tree"() -> (w206:refnum<vi>)
            n90 = call <vilib>:"NT Read and Format Entries as Tree.vi"("Tree Refnum"=w206) -> ()  [unwired: 9 in, 2 out]
          }
          frame "Commands" {
            w215 = u32 5789784 ("Color Box")
            w216 = T27 {"Row"=-1, "Column"=-2} ("Active Cell:Active Cell")
            w218 = T27 {"Row"=-2, "Column"=-2} ("Active Cell:Active Cell")
            n91 = Index Array(array=w219, index=w213) -> (element=w217:u32)
            n92 = Index Array(array=w214, index=w213) -> (element=w212:T26)
            n93 = Unbundle(w212) -> ("Operation"=w211:enum16{"Update", "Clear"})  [unwired: 1 out]
            n94 = local read "Command Selection"() -> (w210:i32)
            n95 = property on="Command Selection" class="MCListbox (strict)"("ActiveCell"=w218, "CellBG"=w217, "ActiveCell"=w216, "CellBG"=w215) -> ()  [unwired: 2 in, 2 out]
            n96 = call <vilib>:"WPI_DashboardUpdate RPC Info.vi"("Operation"=w211) -> ("update"=w209:bool, "commands"=w208:string[][])  [unwired: 9 in]
            n97 = property on="Command Selection" class="MCListbox (strict)"("ItemNames"=w208) -> ()  [unwired: 2 in, 2 out]
            n98 = property on="Command Params" class="Tbl (strict)"("Active Cell"=w218, "Cell BG Color"=w217, "Active Cell"=w216, "Cell BG Color"=w215) -> ()  [unwired: 2 in, 2 out]
            n99 = call <vilib>:"WPI_DashboardUpdate Command Params.vi"("Update"=w209, "NewVal"=w210, "Commands"=w208, "Param Tbl"=w207) -> ()  [unwired: 7 in, 1 out]
          }
        }
        n100 = case shown="\"\"" w194 {
          tunnel: "/TestMode/TestProgress" ("Name") -> [w221 _]
          tunnel: "/TestMode/TestProgressText" ("Name") -> [w220 _]
          frame Default {
            n101 = call <vilib>:"NT Read Number.vi"("Name"=w221) -> ("Numeric"=w222:dbl)  [unwired: 9 in, 1 out]
            n102 = call <vilib>:"NT Read String.vi"("Name"=w220) -> ("String"=w223:string)  [unwired: 9 in, 1 out]
            n103 = Bundle("Numeric"=w222, "String"=w223) -> (→"Progress":cluster{"Numeric":dbl, "String":string})  [unwired: 1 in]
          }
          frame "" {
            n104 = property on="Progress" class="Clust (strict)"("Visible"=FALSE) -> ()  [unwired: 2 in, 2 out]
            n105 = local write "Test Name"(u16 0) -> ()
          }
        }
        n106 = call <vilib>:"Connextion Info.vi"() -> ("Connected"=→"NT Connection":bool)  [unwired: 10 in, 1 out]
      }
      event "Test Tree": Value Change {
        # "Show appropriate\ncontrols"
        n107 = event-data() -> ("CtlRef"=w232:refnum<vi>, "NewVal"=w230:string)  [unwired: 1 in]
        n108 = call <vilib>:"WPI_UtilitiesGetTreeIOName.vi"("NewVal"=w230, "TreeControl in"=w232) -> ("I/O Name"=w233:string)  [unwired: 9 in]
        n109 = case shown="\"Analog Out\", \"Motor\", \"PWM\"" w233 {
          selector: w233 -> [_ w240 _ w262 w271 _]
          tunnel: w230 -> [_ _ w259 w261 _ w278]
          tunnel: w229 -> [_ _ _ _ _ w277]
          frame Default {
            w235 = FALSE ("Visible")
            w234 = FALSE ("Visible")
            n110 = property on="Motor" class="Clust (strict)"("Visible"=w234) -> ()  [unwired: 2 in, 2 out]
            n111 = property on="Test Ring" class="Ring (strict)"("Visible"=w234) -> ()  [unwired: 2 in, 2 out]
            n112 = property on="Rev/Fwd" class="Clust (strict)"("Visible"=w235) -> ()  [unwired: 2 in, 2 out]
            n113 = property on="On/Off" class="Bool (strict)"("Visible"=w235) -> ()  [unwired: 2 in, 2 out]
            n114 = property on="Test Slider" class="Slide (strict)"("Visible"=w235) -> ()  [unwired: 2 in, 2 out]
          }
          frame "Analog Out", "Motor", "PWM" {
            w241 = FALSE ("Visible")
            n115 = case shown="\"Analog Out\"" w240 {
              tunnel: [1.0 ("Value") -1.0 ("Value") 0.0 ("Value")] -> w239
              tunnel: [255.0 ("Value") 1.0 ("Value") 5.0 ("Value")] -> w238
              tunnel: [128.0 ("Value") 0.0 ("Value") 0.0 ("Value")] -> w237
              tunnel: [64.0 ("Value") 0.5 ("Value") 1.0 ("Value")] -> w236
              frame "PWM" {
              }
              frame "Motor", Default {
              }
              frame "Analog Out" {
              }
            }
            n116 = property on="Motor" class="Clust (strict)"("Visible"=TRUE) -> ()  [unwired: 2 in, 2 out]
            n117 = property on="Value" class="Slide (strict)"("Value"=w237, "Scale.Minimum"=w239, "Scale.Maximum"=w238, "Scale.Increment"=w236) -> ()  [unwired: 2 in, 2 out]
            n118 = property on="On/Off" class="Bool (strict)"("Visible"=w241) -> ()  [unwired: 2 in, 2 out]
            n119 = property on="Test Slider" class="Slide (strict)"("Visible"=w241) -> ()  [unwired: 2 in, 2 out]
            n120 = property on="Test Ring" class="Ring (strict)"("Visible"=w241) -> ()  [unwired: 2 in, 2 out]
            n121 = property on="Rev/Fwd" class="Clust (strict)"("Visible"=w241) -> ()  [unwired: 2 in, 2 out]
          }
          frame "Servo" {
            w257 = FALSE ("Visible")
            n122 = call <vilib>:"NT Read Number.vi"("Name"=w259) -> ("Numeric"=w258:dbl)  [unwired: 9 in, 1 out]
            n123 = property on="Test Slider" class="Slide (strict)"("Visible"=TRUE, "Scale.Maximum"=170.0 ("Scale.Range:Maximum")) -> ()  [unwired: 2 in, 2 out]
            n124 = local write "Test Slider"(w258) -> ()
            n125 = property on="Motor" class="Clust (strict)"("Visible"=w257) -> ()  [unwired: 2 in, 2 out]
            n126 = property on="Rev/Fwd" class="Clust (strict)"("Visible"=w257) -> ()  [unwired: 2 in, 2 out]
            n127 = property on="On/Off" class="Bool (strict)"("Visible"=w257) -> ()  [unwired: 2 in, 2 out]
            n128 = property on="Test Ring" class="Ring (strict)"("Visible"=w257) -> ()  [unwired: 2 in, 2 out]
          }
          frame "Relay", "Solenoid" {
            w260 = FALSE ("Visible")
            n129 = property on="Motor" class="Clust (strict)"("Visible"=w260) -> ()  [unwired: 2 in, 2 out]
            n130 = property on="Test Slider" class="Slide (strict)"("Visible"=w260) -> ()  [unwired: 2 in, 2 out]
            n131 = Search and Replace String(input string=w261, search string="/Value  **", replace string="/Direction") -> (result string=w267:string)  [unwired: 5 in, 3 out]
            n132 = property on="Test Ring" class="Ring (strict)"("Visible"=w260) -> ()  [unwired: 2 in, 2 out]
            n133 = call <vilib>:"NT Read String.vi"("Name"=w267) -> ("String"=w265:string)  [unwired: 9 in, 1 out]
            n134 = Equal?(x="Both directions", y=w265) -> (x = y?=w263:bool)
            n135 = Not(x=w263) -> (.not. x?=w264:bool)
            n136 = property on="Rev/Fwd" class="Clust (strict)"("Visible"=w263) -> ()  [unwired: 2 in, 2 out]
            n137 = property on="On/Off" class="Bool (strict)"("Visible"=w264, "Caption.Text"=w262) -> ()  [unwired: 2 in, 2 out]
          }
          frame "Compressor", "Digital Out" {
            w270 = FALSE ("Visible")
            # "Get direction and finish"
            n138 = property on="Motor" class="Clust (strict)"("Visible"=w270) -> ()  [unwired: 2 in, 2 out]
            n139 = property on="Test Slider" class="Slide (strict)"("Visible"=w270) -> ()  [unwired: 2 in, 2 out]
            n140 = property on="Test Ring" class="Ring (strict)"("Visible"=w270) -> ()  [unwired: 2 in, 2 out]
            n141 = property on="On/Off" class="Bool (strict)"("Visible"=TRUE, "Caption.Text"=w271) -> ()  [unwired: 2 in, 2 out]
            n142 = property on="Rev/Fwd" class="Clust (strict)"("Visible"=FALSE) -> ()  [unwired: 2 in, 2 out]
          }
          frame "Camera" {
            n143 = call <vilib>:"Get Last Path Segment.vi"("String in"=w278) -> ("String out"=w279:string)  [unwired: 10 in]
            n144 = property on="On/Off" class="Bool (strict)"("Visible"=FALSE) -> ()  [unwired: 2 in, 2 out]
            n145 = property on="Motor" class="Clust (strict)"("Visible"=FALSE) -> ()  [unwired: 2 in, 2 out]
            n146 = property on="Rev/Fwd" class="Clust (strict)"("Visible"=FALSE) -> ()  [unwired: 2 in, 2 out]
            n147 = case shown="\"White Balance  **\"" w279 {
              tunnel: w278 -> [w285 w294 w303 w312 w321 _ w327]
              tunnel: w277 -> [w283 w291 w300 w309 w318 _ _]
              frame "Size  **" {
                n148 = Index Array(array=w283) -> (element=w282:cluster{string[]})  [unwired: 1 in]
                n149 = call <vilib>:"NT Read String.vi"("Name"=w285) -> ("String"=w284:string)  [unwired: 9 in, 1 out]
                n150 = Unbundle(w282) -> (w280:string[])
                n151 = Match First String(2:w280, 3:w284) -> (0:w281:i32)  [unwired: 1 out]
                n152 = property on="Test Ring" class="Ring (strict)"("Value"=w281, "Strings []"=w280) -> ()  [unwired: 2 in, 2 out]
                n153 = property on="Test Ring" class="Ring (strict)"("Visible"=TRUE) -> ()  [unwired: 2 in, 2 out]
                n154 = property on="Test Slider" class="Slide (strict)"("Visible"=FALSE) -> ()  [unwired: 2 in, 2 out]
              }
              frame "White Balance  **" {
                n155 = Index Array(array=w291, index=1) -> (element=w292:cluster{string[]})
                n156 = call <vilib>:"NT Read String.vi"("Name"=w294) -> ("String"=w293:string)  [unwired: 9 in, 1 out]
                n157 = Unbundle(w292) -> (w289:string[])
                n158 = Match First String(2:w289, 3:w293) -> (0:w288:i32)  [unwired: 1 out]
                n159 = property on="Test Ring" class="Ring (strict)"("Value"=w288, "Strings []"=w289) -> ()  [unwired: 2 in, 2 out]
                n160 = property on="Test Ring" class="Ring (strict)"("Visible"=TRUE) -> ()  [unwired: 2 in, 2 out]
                n161 = property on="Test Slider" class="Slide (strict)"("Visible"=FALSE) -> ()  [unwired: 2 in, 2 out]
              }
              frame "Exposure  **" {
                n162 = Index Array(array=w300, index=2) -> (element=w301:cluster{string[]})
                n163 = call <vilib>:"NT Read String.vi"("Name"=w303) -> ("String"=w302:string)  [unwired: 9 in, 1 out]
                n164 = Unbundle(w301) -> (w297:string[])
                n165 = Match First String(2:w297, 3:w302) -> (0:w298:i32)  [unwired: 1 out]
                n166 = property on="Test Ring" class="Ring (strict)"("Value"=w298, "Strings []"=w297) -> ()  [unwired: 2 in, 2 out]
                n167 = property on="Test Ring" class="Ring (strict)"("Visible"=TRUE) -> ()  [unwired: 2 in, 2 out]
                n168 = property on="Test Slider" class="Slide (strict)"("Visible"=FALSE) -> ()  [unwired: 2 in, 2 out]
              }
              frame "Exposure Priority  **" {
                n169 = Index Array(array=w309, index=3) -> (element=w310:cluster{string[]})
                n170 = call <vilib>:"NT Read String.vi"("Name"=w312) -> ("String"=w311:string)  [unwired: 9 in, 1 out]
                n171 = Unbundle(w310) -> (w306:string[])
                n172 = Match First String(2:w306, 3:w311) -> (0:w307:i32)  [unwired: 1 out]
                n173 = property on="Test Ring" class="Ring (strict)"("Value"=w307, "Strings []"=w306) -> ()  [unwired: 2 in, 2 out]
                n174 = property on="Test Ring" class="Ring (strict)"("Visible"=TRUE) -> ()  [unwired: 2 in, 2 out]
                n175 = property on="Test Slider" class="Slide (strict)"("Visible"=FALSE) -> ()  [unwired: 2 in, 2 out]
              }
              frame "Color Enable  **" {
                n176 = Index Array(array=w318, index=4) -> (element=w319:cluster{string[]})
                n177 = call <vilib>:"NT Read String.vi"("Name"=w321) -> ("String"=w320:string)  [unwired: 9 in, 1 out]
                n178 = Unbundle(w319) -> (w315:string[])
                n179 = Match First String(2:w315, 3:w320) -> (0:w316:i32)  [unwired: 1 out]
                n180 = property on="Test Ring" class="Ring (strict)"("Value"=w316, "Strings []"=w315) -> ()  [unwired: 2 in, 2 out]
                n181 = property on="Test Ring" class="Ring (strict)"("Visible"=TRUE) -> ()  [unwired: 2 in, 2 out]
                n182 = property on="Test Slider" class="Slide (strict)"("Visible"=FALSE) -> ()  [unwired: 2 in, 2 out]
              }
              frame Default {
                n183 = property on="Test Ring" class="Ring (strict)"("Visible"=FALSE) -> ()  [unwired: 2 in, 2 out]
                n184 = property on="Test Slider" class="Slide (strict)"("Visible"=FALSE) -> ()  [unwired: 2 in, 2 out]
              }
              frame "Brightness  **", "Color Level  **", "Compression  **", "FPS  **", "Sharpness  **" {
                n185 = call <vilib>:"NT Read Number.vi"("Name"=w327) -> ("Numeric"=w326:dbl)  [unwired: 9 in, 1 out]
                n186 = local write "Test Slider"(w326) -> ()
                n187 = property on="Test Slider" class="Slide (strict)"("Visible"=TRUE, "Scale.Maximum"=100.0 ("Scale.Range:Maximum")) -> ()  [unwired: 2 in, 2 out]
                n188 = property on="Test Ring" class="Ring (strict)"("Visible"=FALSE) -> ()  [unwired: 2 in, 2 out]
              }
            }
          }
        }
        n189 = property on="Progress" class="Clust (strict)"("Visible"=FALSE) -> ()  [unwired: 2 in, 2 out]
      }
      event "Test Name": Mouse Enter {
        # "Populate the ring with the list of tests"
        n190 = event-data() -> ()  [unwired: 1 in, 1 out]
        n191 = call <vilib>:"NT Read String Array.vi"("Name"="/TestMode/TestList") -> ("String Array"=w336:string[])  [unwired: 9 in, 1 out]
        n192 = Build Array (concatenate)("Select the test to run...", w336) -> (w335:string[])
        n193 = property on="Test Name" class="Ring (strict)"("Strings []"=w335) -> ()  [unwired: 2 in, 2 out]
      }
      event "Test Name": Value Change {
        w339 = FALSE ("Visible")
        # "Tell the robot the test name to run"
        n194 = event-data() -> ("NewVal"=w343:u16)  [unwired: 1 in]
        n195 = property on="Test Name" class="Ring (strict)"() -> ("Strings []"=w344:string[])  [unwired: 2 in, 2 out]
        n196 = local write "Progress"(T6 {"Test Progress"=0, "Test Progress Text"=""} ("Progress")) -> ()
        n197 = Index Array(array=w344, index=w343) -> (element=w342:string)
        n198 = call <vilib>:"NT Write String.vi"("String"=w342, "Name"="/TestMode/TestName") -> ()  [unwired: 9 in, 1 out]
        n199 = property on="Progress" class="Clust (strict)"("Visible"=TRUE) -> ()  [unwired: 2 in, 2 out]
        n200 = property on="Motor" class="Clust (strict)"("Visible"=w339) -> ()  [unwired: 2 in, 2 out]
        n201 = property on="Test Slider" class="Slide (strict)"("Visible"=w339) -> ()  [unwired: 2 in, 2 out]
        n202 = property on="On/Off" class="Bool (strict)"("Visible"=w339) -> ()  [unwired: 2 in, 2 out]
        n203 = property on="Rev/Fwd" class="Clust (strict)"("Visible"=w339) -> ()  [unwired: 2 in, 2 out]
        n204 = property on="Test Ring" class="Ring (strict)"("Visible"=w339) -> ()  [unwired: 2 in, 2 out]
      }
      event "Command Selection": Value Change {
        # "Get the params and show in table"
        n205 = event-data() -> ("NewVal"=w349:i32)  [unwired: 1 in]
        n206 = property on="Command Selection" class="MCListbox (strict)"() -> ("ItemNames"=w347:string[][])  [unwired: 2 in, 2 out]
        n207 = call <vilib>:"WPI_DashboardUpdate Command Params.vi"("NewVal"=w349, "Commands"=w347, "Param Tbl"=w348) -> ()  [unwired: 8 in, 1 out]
      }
      event "Execute Command": Value Change {
        # "Started one, Unique ID holds\nresponse"
        n208 = event-data() -> ()  [unwired: 1 in, 1 out]
        n209 = property on="Command Selection" class="MCListbox (strict)"() -> ("ItemNames"=w361:string[][])  [unwired: 2 in, 2 out]
        n210 = Index Array(array=w361, index (row)="Command Selection", index (col)=0) -> (element=w359:string)
        n211 = call <vilib>:"Invoke Commands.vi"("Command Params"="Command Params", "Function Name"=w359) -> ("Params"=w355:u8, "Started"=w354:bool)  [unwired: 7 in, 1 out]
        n212 = Array Subset(array="Command Params", length (row)=w355) -> (w356:string[][])  [unwired: 3 in]
        n213 = Select(t="Executing" ("Cmd Status"), s=w354, f="" ("Cmd Status")) -> (s? t:f=→"Cmd Status":string)
      }
      event "Command Selection": Double Click {
        n214 = event-data() -> ("Row"=w371:i32)  [unwired: 1 in]
        n215 = property on="Command Selection" class="MCListbox (strict)"() -> ("ItemNames"=w374:string[][])  [unwired: 2 in, 2 out]
        n216 = local read "Command Params"() -> (w369:string[][])
        n217 = Index Array(array=w374, index (row)=w371, index (col)=0) -> (element=w372:string)
        n218 = call <vilib>:"Invoke Commands.vi"("Command Params"=w369, "Function Name"=w372) -> ("Params"=w368:u8, "Started"=w363:bool)  [unwired: 7 in, 1 out]
        n219 = Array Subset(array=w369, length (row)=w368) -> (w367:string[][])  [unwired: 3 in]
        n220 = Select(t="Executing" ("Cmd Status"), s=w363, f="" ("Cmd Status")) -> (s? t:f=w364:string)
        n221 = local write "Cmd Status"(w364) -> ()
      }
      event "CheckList": Double Click {
        # "Shift clears all"
        # "Update symbols on the listbox"
        n222 = event-data() -> ("PlatMods.Shift"=w377:bool, "Row"=w379:i32)  [unwired: 1 in]
        n223 = case shown="True" w377 {
          tunnel: w379 -> [w383 _]
          tunnel: 1 -> [w382 _]
          frame False {
            n224 = property on="CheckList" class="LstBox (strict)"() -> ("Item Symbols"=w381:i32[])  [unwired: 2 in, 2 out]
            n225 = Replace Array Subset(array=w381, new element=w382, index=w383) -> (w380:i32[])
            n226 = property on="CheckList" class="LstBox (strict)"("Item Symbols"=w380) -> ()  [unwired: 2 in, 2 out]
          }
          frame True {
            w384 = 0 ("Top Row")
            n227 = property on="CheckList" class="LstBox (strict)"() -> ("Number of Rows"=w386:u32)  [unwired: 2 in, 2 out]
            n228 = Initialize Array(0, w386) -> (w385:i32[])
            n229 = property on="CheckList" class="LstBox (strict)"("Top Row"=w384, "Value"=w384, "Item Symbols"=w385) -> ()  [unwired: 2 in, 2 out]
          }
        }
      }
      event "CheckList": Key Down {
        # "Update symbols on the listbox\nLeft and right keys check and uncheck"
        n230 = event-data() -> ("VKey"=w391:T25)  [unwired: 1 in]
        n231 = case shown="\"Left\", \"Right\"" w391 {
          selector: w391 -> [w396 _]
          tunnel: eventvkey."Left" ("VKey") -> [w394 _]
          frame "Left", "Right" {
            n232 = Equal?(x=w394, y=w396) -> (x = y?=w395:bool)
            n233 = Select(t=0, s=w395, f=1) -> (s? t:f=w397:i32)
            n234 = property on="CheckList" class="LstBox (strict)"() -> ("Item Symbols"=w400:i32[])  [unwired: 2 in, 2 out]
            n235 = Replace Array Subset(array=w400, new element=w397, index="CheckList") -> (w399:i32[])
            n236 = property on="CheckList" class="LstBox (strict)"("Item Symbols"=w399) -> ()  [unwired: 2 in, 2 out]
          }
          frame Default {
          }
        }
      }
      event "Motor.Enable": Value Change {
        # "When the test mode otor enable helper is set, update that\ntree row item's value"
        n237 = event-data() -> ("NewVal"=w407:bool)  [unwired: 1 in]
        n238 = Unbundle("Motor") -> ("Value"=w406:dbl)  [unwired: 1 out]
        n239 = Select(t=w406, s=w407, f=0.0) -> (s? t:f=w404:dbl)
        n240 = call <vilib>:"NT Write Number.vi"("Numeric"=w404, "Name"=w403) -> ()  [unwired: 9 in, 1 out]
      }
      event "Test Slider": Value Change {
        # "When the test mode slider helper is set, update that\ntree row item's value"
        n241 = event-data() -> ("NewVal"=w411:dbl)  [unwired: 1 in]
        n242 = call <vilib>:"NT Write Number.vi"("Numeric"=w411, "Name"=w412) -> ()  [unwired: 9 in, 1 out]
      }
      event "On/Off": Value Change {
        # "When the test mode on/off helper value is set, update that\ntree row item's value"
        n243 = event-data() -> ("NewVal"=w417:bool)  [unwired: 1 in]
        n244 = Boolean To (0,1)(Boolean=w417) -> (0, 1=w416:i16)
        n245 = call <vilib>:"NT Write Number.vi"("Numeric"=w416, "Name"=w415) -> ()  [unwired: 9 in, 1 out]
      }
      event "Rev/Fwd": Value Change {
        # "When the test mode helper value for relays is set, update that\ntree row item's value"
        n246 = event-data() -> ("NewVal.Forward"=w426:bool, "NewVal.Reverse"=w425:bool)  [unwired: 1 in]
        n247 = Boolean To (0,1)(Boolean=w426) -> (0, 1=w422:i16)
        n248 = Boolean To (0,1)(Boolean=w425) -> (0, 1=w424:i16)
        n249 = Negate(x=w424) -> (-x=w423:i16)
        n250 = Add(x=w422, y=w423) -> (x+y=w421:i16)
        n251 = call <vilib>:"NT Write Number.vi"("Numeric"=w421, "Name"=w420) -> ()  [unwired: 9 in, 1 out]
      }
      event "Test Ring": Value Change {
        # "When a test mode helper value is selected from the ring,\nset the tree item's variable to the string value"
        n252 = event-data() -> ("NewVal"=w431:u16)  [unwired: 1 in]
        n253 = property on="Test Ring" class="Ring (strict)"() -> ("Strings []"=w432:string[])  [unwired: 2 in, 2 out]
        n254 = Index Array(array=w432, index=w431) -> (element=w430:string)
        n255 = call <vilib>:"NT Write String.vi"("String"=w430, "Name"=w429) -> ()  [unwired: 9 in, 1 out]
      }
      event Panel Close {
        # "Playback window has been closed, abort"
        n256 = event-data() -> ()  [unwired: 1 in, 4 out]
        n257 = global write "WPI_DashboardLogging Global.vi" "Recording"(enum32{"Stop", "Record", "Playback"}."Stop" ("Rec Mode")) -> ()
      }
      event Panel Close {
        # "Abort playback window and ourself"
        n258 = event-data() -> ()  [unwired: 1 in, 4 out]
        n259 = invoke class="VI" method="FP.Close"() -> (reference out=w439:refnum<vi>)  [unwired: 3 in, 2 out]
        n260 = invoke class="VI" method="Abort VI"(reference=w439) -> (error out=w438:errorcluster)  [unwired: 2 in, 2 out]
        n261 = invoke class="VI" method="Abort VI"(error in=w438) -> ()  [unwired: 2 in, 3 out]
      }
      event User Event {
        n262 = event-data() -> ("IDs"=w447:cluster{"RPC field ID":u16, "Unique ID":u16}, "String"=w446:string)  [unwired: 1 in]
        n263 = Bundle("IDs"=w447, "String"=w446) -> (w445:T9)  [unwired: 1 in]
        n264 = call <vilib>:"Retrieve RPC Response.vi"("RPC Response"=w445) -> ("Output"=w442:string[][])  [unwired: 10 in]
        n265 = Build Array (concatenate)(w440, w442) -> (w441:string[][])
        n266 = local write "Command Params"(w441) -> ()
        n267 = local write "Cmd Status"("" ("Cmd Status")) -> ()
      }
      event "Tree": Double Click {
        n268 = event-data() -> ("PlatMods"=w451:T28, "Tag"=w450:string)  [unwired: 1 in]
        n269 = Unbundle(w451) -> ("Shift"=w449:bool)  [unwired: 4 out]
        n270 = Not(x=w449) -> (.not. x?=w448:bool)
        n271 = call <vilib>:"NT Update Persistence.vi"("Persistence"=w448, "Name"=w450) -> ()  [unwired: 9 in, 1 out]
      }
    }
  }
  n272 = local write "Dashboard Tab"(T1."Garnet Squadron" ("Dashboard Tab")) -> ()
  n273 = property on="On/Off" class="Bool (strict)"("Visible"=w16) -> ()  [unwired: 2 in, 2 out]
  n274 = property on="Motor" class="Clust (strict)"("Visible"=w16) -> ()  [unwired: 2 in, 2 out]
  n275 = property on="Progress" class="Clust (strict)"("Visible"=w16) -> ()  [unwired: 2 in, 2 out]
  n276 = property on="Test Ring" class="Ring (strict)"("Visible"=w16) -> ()  [unwired: 2 in, 2 out]
  n277 = property on="Rev/Fwd" class="Clust (strict)"("Visible"=w16) -> ()  [unwired: 2 in, 2 out]
  n278 = local write "DB Camera Config"(w16) -> ()
  n279 = while {
    tunnel: u16 1741 ("timeout ms (25000)") -> [w455]
    stop <- FALSE stop-if-true
    n280 = TCP Create Listener(10:w455) -> (0:w454:errorcluster, 3:w456:refnum<k5>)  [unwired: 4 in, 1 out]
    n281 = case shown="No Error" w454 {
      selector: w454 -> [w458 _]
      tunnel: w456 -> [w459 _]
      frame No Error {
        n282 = while {
          tunnel: w459 -> [w462]
          tunnel: w458 -> [w461]
          stop <- FALSE stop-if-true
          n283 = TCP Wait On Listener(8:w461, 11:w462) -> (0:w463:errorcluster, 4:w464:refnum<k5>)  [unwired: 2 in, 3 out]
          n284 = local write "TCP"(w464) -> ()
          n285 = case shown="No Error" w463 {
            frame No Error {
            }
            frame Error {
              n286 = Wait (ms)(milliseconds to wait=u32 1000) -> ()  [unwired: 1 out]
            }
          }
        }
      }
      frame Error {
        n287 = Wait (ms)(milliseconds to wait=u32 1000) -> ()  [unwired: 1 out]
      }
    }
  }
  n288 = local write "Command Params"(string[][] [] ("Command Params")) -> ()
  n289 = local write "Command Selection"(u16 0 ("milliseconds to wait")) -> ()
